vi "Write File.vi"(8 "error in (no error)":errorcluster, 11 "Data.ITX in":refnum<class "Data.ITX.lvclass">) -> (0 "error out":errorcluster, 3 "Data.ITX out":refnum<class "Data.ITX.lvclass">)   [LabVIEW 2016, in "Data.ITX.lvclass"]
uses:
  Data.ITX.lvclass
  Users/patrickirvin/Documents/GitHub/LV-to-ITX/src/Data/Data.lvclass
  Data/Data.lvclass/Data.ctl
  Data/Data.lvclass
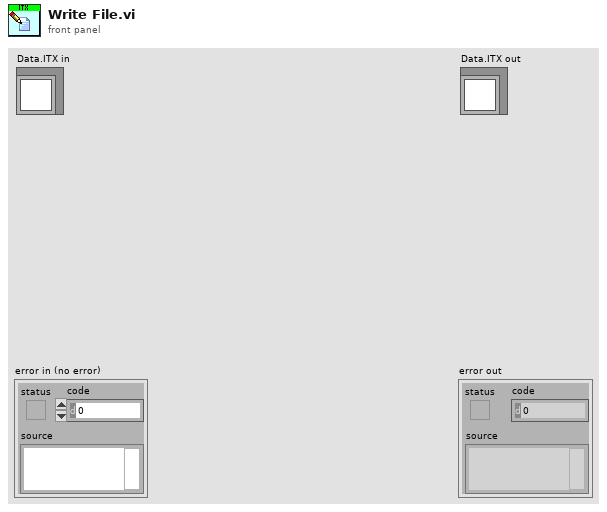
[diagram p1: front panel]
types:
  T1 = typedef "Data.lvclass/Dictionary--cluster.ctl" = cluster{"key":string, "value":variant}
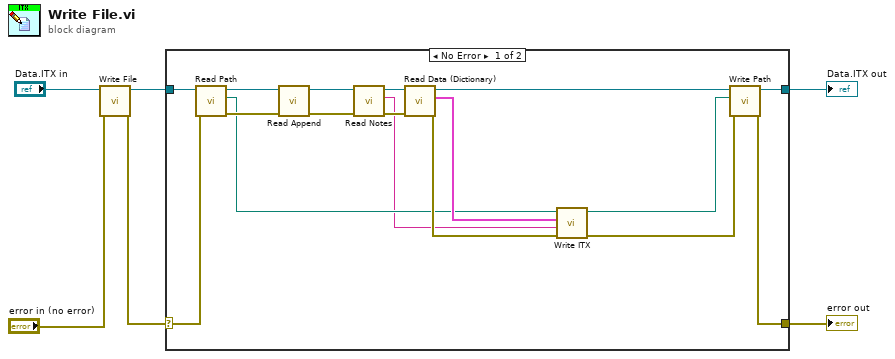
[diagram p0: block diagram]
diagram:
  n1 = call-parent "Write File.vi"("error in (no error)"="error in (no error)", "Data in"="Data.ITX in") -> ("error out"=w3:errorcluster, "Data out"=w5:refnum<class "Data.ITX.lvclass">)  [unwired: 8 in]
  n2 = case shown="No Error" w3 {
    selector: w3 -> [w20 w25]
    tunnel: [w17 w25] -> w1
    tunnel: w5 -> [w21 w24]
    tunnel: [w18 w24] -> w2
    frame No Error {
      n3 = call "Read Path.vi"("error in (no error)"=w20, "Data Save"=w21) -> ("error out"=w15:errorcluster, "Path"=w10:path, "Data Save out"=w16:refnum<class "Data.ITX.lvclass">)  [unwired: 7 in]
      n4 = call "Read Append.vi"("error in (no error)"=w15, "Data in"=w16) -> ("error out"=w13:errorcluster, "Data out"=w14:refnum<class "Data.ITX.lvclass">)  [unwired: 7 in, 1 out]
      n5 = call "Read Notes.vi"("error in (no error)"=w13, "Data Save"=w14) -> ("error out"=w22:errorcluster, "Comments"=w9:string, "Data Save out"=w23:refnum<class "Data.ITX.lvclass">)  [unwired: 7 in]
      n6 = call "Read Data (Dictionary).vi"("error in (no error)"=w22, "Data Save"=w23) -> ("error out"=w11:errorcluster, "Data (Dictionary)"=w12:T1[], "Data Save out"=w19:refnum<class "Data.ITX.lvclass">)  [unwired: 7 in]
      n7 = call "Write ITX.vi"("error in"=w11, "Notes"=w9, "Data (Dictionary)"=w12, "filename"=w10) -> ("error out"=w8:errorcluster, "file"=w7:path)  [unwired: 6 in]
      n8 = call "Write Path.vi"("error in (no error)"=w8, "Path"=w7, "Data Save"=w19) -> ("error out"=w17:errorcluster, "Data Save out"=w18:refnum<class "Data.ITX.lvclass">)  [unwired: 7 in]
    }
    frame Error {
    }
  }
  "error out" <- w1
  "Data.ITX out" <- w2
